vi "Target Sender.vi"() -> ()   [LabVIEW 2013]
doc: "This example demonstrates how to handle communications with multiple servers at once. Each server will ping the host over UDP in order to establish a TCP connection. Once a TCP connection is established, the server and client work in a typical command based fashion. Instead of a single server to communicate with though, the client must handle multiple connections."
uses:
  vi.lib/NI/STM/TCP/TCP Connection Info.ctl
  vi.lib/NI/STM/SubVIs/MetaDataElement.ctl
  Target SubVIs/ClientConnectionStates.ctl
  vi.lib/NI/STM/TCP/TCP Read Options.ctl
  vi.lib/NI/STM/UDP/Set Meta Data (UDP Ref).vi
  vi.lib/NI/STM/UDP/Get Connection Reference (UDP).vi
  vi.lib/NI/STM/TCP/Set Meta Data (TCP Ref).vi
  vi.lib/NI/STM/TCP/Get Connection Reference (TCP).vi
  vi.lib/NI/STM/TCP/Write Message (TCP).vi
  vi.lib/NI/STM/UDP/Write Message (UDP).vi
  vi.lib/NI/STM/TCP/Read Meta Data (TCP Clst).vi
  vi.lib/NI/STM/TCP/Read Message (TCP).vi
  vi.lib/NI/STM/NI STM.lvlib
panel:
  out "Connection Info":T1
  out "Connected":bool
  out "Host IP Address":string
  out "Waveform Graph":dbl[](graph)
  out "My IP Address":string
  out "error  out":errorcluster
  in  "stop":bool
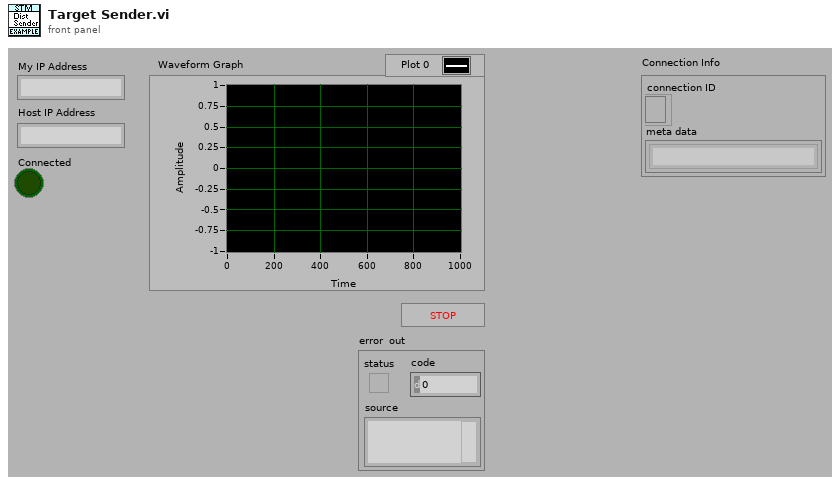
[diagram p1: front panel]
types:
  T1 = typedef "NI STM.lvlib/TCP Connection Info.ctl" = cluster{"connection ID":refnum<k5>, "meta data":T2[]}
  T2 = typedef "NI STM.lvlib/MetaDataElement.ctl" = string
  T3 = typedef "ClientConnectionStates.ctl" = enum16{"Init", "Ping Host", "Wait for Host Connection", "Read Meta Data", "Receive Commands", "Close Connection", "Shutdown"}
  T4 = typedef "NI STM.lvlib/TCP Read Options.ctl" = cluster{"ignore timeout error":bool, "timeout ms (1000)":i32}
  T5 = typedef "NI STM.lvlib/UDP Connection Info.ctl" = cluster{"connection ID":refnum<k16>, "meta data":T2[]}
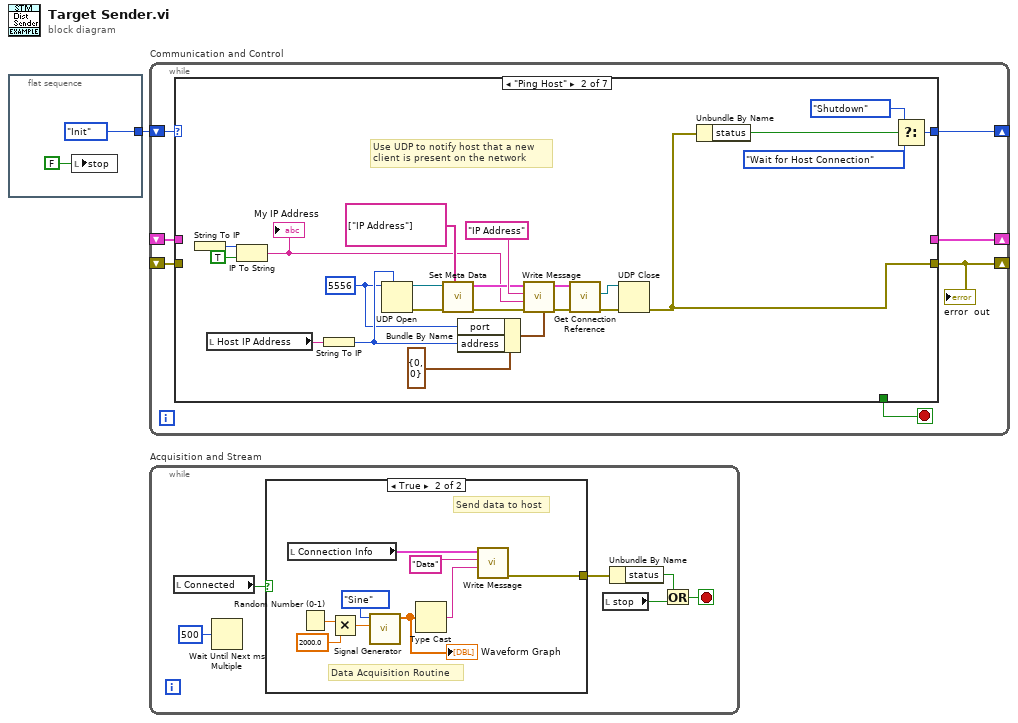
[diagram p0: block diagram]
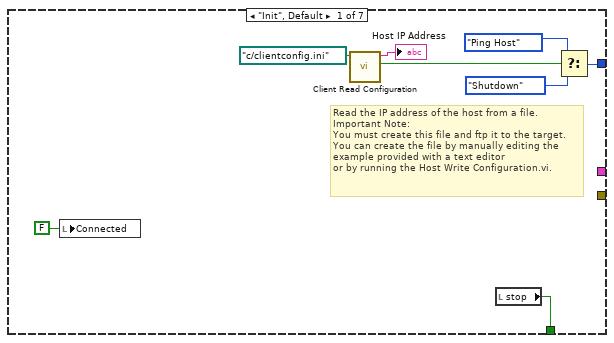
[diagram p2: hidden frame]
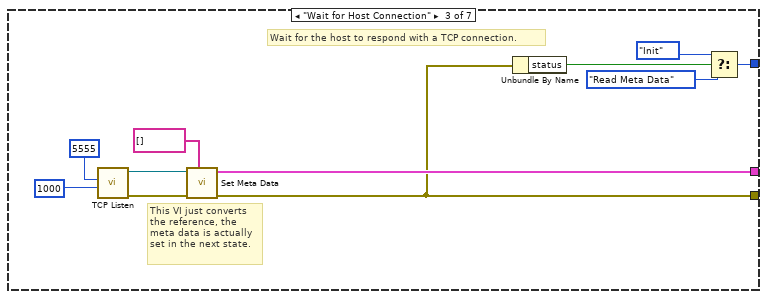
[diagram p3: hidden frame]
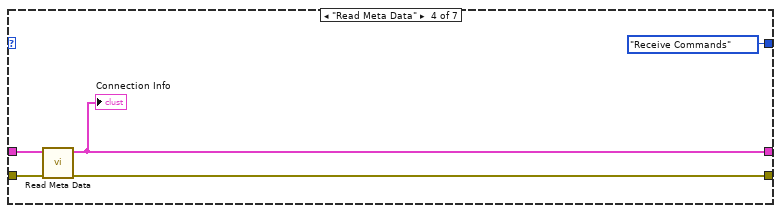
[diagram p4: hidden frame]
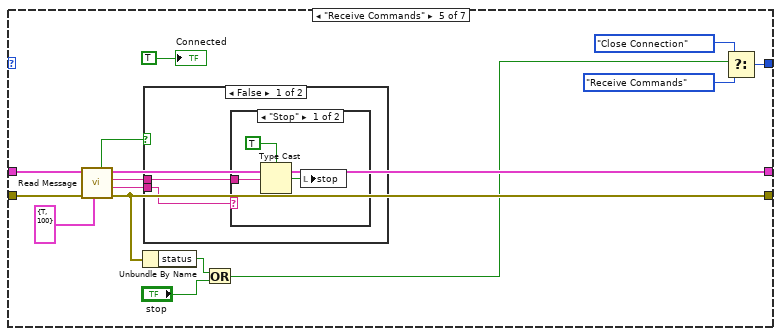
[diagram p5: hidden frame]
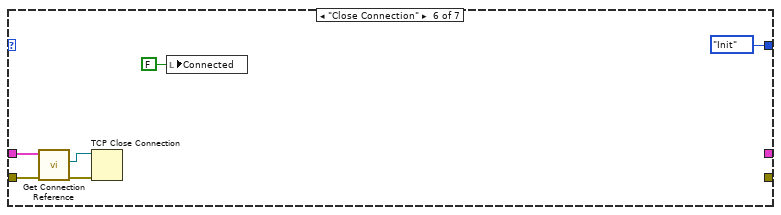
[diagram p8: hidden frame]
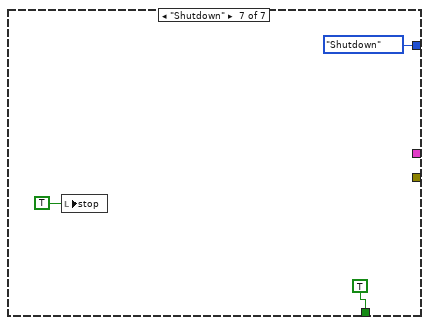
[diagram p9: hidden frame]
diagram:
  n1 = flat-sequence {
    tunnel: [ClientConnectionStates."Init" ("Connection States")] -> w1
    frame #0 {
      n2 = local write "stop"(FALSE ("stop")) -> ()
    }
  }
  n3 = while "Communication and Control" {
    shift-right: [w9] -> _
    shift-left: _ -> [w7]
    shift-right: [w8] -> _
    shift-left: w1 -> [w10]
    shift-right: [w5] -> _
    shift-left: _ -> [w6]
    stop <- w4 stop-if-true
    n4 = case shown="\"Ping Host\"" w10 {
      tunnel: [_ _ w44 w56 w70 _ _] -> w9
      tunnel: [w15 w37 w47 ClientConnectionStates."Receive Commands" ("Connection States") w60 ClientConnectionStates."Init" ("Connection States") ClientConnectionStates."Shutdown" ("Connection States")] -> w8
      tunnel: w7 -> [_ _ _ w57 w72 w79 _]
      tunnel: [_ w40 w43 w54 w69 _ _] -> w5
      tunnel: w6 -> [_ _ _ w55 w71 w81 _]
      tunnel: [w14 _ _ _ _ _ TRUE] -> w4
      frame "Init", Default {
        # "Read the IP address of the host from a file.\nImportant Note:\nYou must create this file and ftp it to the target.\nYou can create the file by manually editing the\nexample provided with a text editor\nor by running the Host Write Configuration.vi."
        n5 = local write "Connected"(FALSE ("Connected")) -> ()
        n6 = call "Client Read Configuration.vi"("configuration file path"=path "c:/clientconfig.ini") -> ("valid data"=w13:bool, "Host IP Address"=→"Host IP Address":string)  [unwired: 8 in, 1 out]
        n7 = local read "stop"() -> (w14:bool)
        n8 = Select(t=ClientConnectionStates."Ping Host" ("Connection States"), s=w13, f=ClientConnectionStates."Shutdown" ("Connection States")) -> (s? t:f=w15:T3)
      }
      frame "Ping Host" {
        w29 = u16 5556 ("port")
        # "Use UDP to notify host that a new client is present on the network"
        n9 = String To IP() -> (0:w20:u32)  [unwired: 1 out]
        n10 = local read "Host IP Address"() -> (w41:string)
        n11 = IP To String(1:TRUE ("dot notation? (F)"), 2:w20) -> (0:w19:string)
        "My IP Address" <- w19
        n12 = String To IP(1:w41) -> (0:w30:u32)
        n13 = UDP Open(7:w30, 11:w29) -> (port=w32:refnum<k16>, 0:w34:errorcluster)  [unwired: 3 in, 1 out]
        n14 = call-poly "Set Meta Data.vi"("meta data"=T2[] ["IP Address"] ("Meta data"), "error in"=w34, "connection ID"=w32) -> ("error out"=w33:errorcluster, "connection info out"=w31:T5)  [unwired: 7 in]
        n15 = Bundle By Name(cluster=cluster{"address":u32, "port":u16} {"address"=0, "port"=0} ("Address"), "port"=w29, "address"=w30) -> (w27:cluster{"address":u32, "port":u16})
        n16 = call-poly "Write Message.vi"("address"=w27, "error in"=w33, "data"=w19, "name"="IP Address" ("Name"), "connection info in"=w31) -> ("error out"=w26:errorcluster, "connection info out"=w24:T5)  [unwired: 5 in]
        n17 = call-poly "Get Connection Reference.vi"("error in"=w26, "connection info in"=w24) -> ("error out"=w25:errorcluster, "connection ID"=w23:refnum<k16>)  [unwired: 7 in, 1 out]
        n18 = UDP Close(connection ID=w23, 8:w25) -> (error out=w40:errorcluster)  [unwired: 1 out]
        n19 = Unbundle By Name(w40) -> ("status"=w38:bool)
        n20 = Select(t=ClientConnectionStates."Shutdown" ("Connection States"), s=w38, f=ClientConnectionStates."Wait for Host Connection" ("Connection States")) -> (s? t:f=w37:T3)
      }
      frame "Wait for Host Connection" {
        # "This VI just converts \nthe reference, the \nmeta data is actually \nset in the next state."
        # "Wait for the host to respond with a TCP connection."
        n21 = call <vilib>:"TCP Listen.vi"("timeout ms (wait forever: -1)"=1000, "port"=u16 5555) -> ("error out"=w45:errorcluster, "connection ID"=w46:refnum<k5>)  [unwired: 5 in, 3 out]
        n22 = call-poly "Set Meta Data.vi"("meta data"=T2[] [] ("Meta data"), "error in"=w45, "connection ID"=w46) -> ("error out"=w43:errorcluster, "connection info out"=w44:T1)  [unwired: 7 in]
        n23 = Unbundle By Name(w43) -> ("status"=w50:bool)
        n24 = Select(t=ClientConnectionStates."Init" ("Connection States"), s=w50, f=ClientConnectionStates."Read Meta Data" ("Connection States")) -> (s? t:f=w47:T3)
      }
      frame "Read Meta Data" {
        n25 = call-poly "Read Meta Data.vi"("error in"=w55, "connection info in"=w57) -> ("error out"=w54:errorcluster, "connection info out"=w56:T1)  [unwired: 7 in, 1 out]
        "Connection Info" <- w56
      }
      frame "Receive Commands" {
        n26 = call-poly "Read Message.vi"("options"=T4 {"ignore timeout error"=TRUE, "timeout ms (1000)"=100} ("Options"), "error in"=w71, "connection info in"=w72) -> ("error out"=w69:errorcluster, "name"=w66:T2, "data string"=w65:string, "connection info out"=w70:T1, "timed out?"=w64:bool)  [unwired: 3 in, 1 out]
        n27 = Unbundle By Name(w69) -> ("status"=w68:bool)
        n28 = case shown="False" w64 {
          tunnel: w66 -> [w73 _]
          tunnel: w65 -> [w74 _]
          frame False {
            n29 = case shown="\"Stop\"" w73 {
              tunnel: w74 -> [w77 _]
              frame "Stop" {
                n30 = Type Cast(type=TRUE, x=w77) -> (*(type *) &x=w76:bool)
                n31 = local write "stop"(w76) -> ()
              }
              frame Default {
              }
            }
          }
          frame True {
          }
        }
        n32 = Or(x=w68, y="stop") -> (x .or. y?=w63:bool)
        n33 = Select(t=ClientConnectionStates."Close Connection" ("Connection States"), s=w63, f=ClientConnectionStates."Receive Commands" ("Connection States")) -> (s? t:f=w60:T3)
        "Connected" <- TRUE
      }
      frame "Close Connection" {
        n34 = call-poly "Get Connection Reference.vi"("error in"=w81, "connection info in"=w79) -> ("error out"=w78:errorcluster, "connection ID out"=w80:refnum<k5>)  [unwired: 7 in, 1 out]
        n35 = TCP Close Connection(connection ID=w80, error in (no error)=w78) -> ()  [unwired: 1 in, 2 out]
        n36 = local write "Connected"(FALSE ("Connected")) -> ()
      }
      frame "Shutdown" {
        n37 = local write "stop"(TRUE ("stop")) -> ()
      }
    }
    "error  out" <- w5
  }
  n38 = while "Acquisition and Stream" {
    stop <- w92 stop-if-true
    n39 = local read "Connected"() -> (w87:bool)
    n40 = Wait Until Next ms Multiple(millisecond multiple=u32 500) -> ()  [unwired: 1 out]
    n41 = case shown="True" w87 {
      tunnel: [_ w100] -> w88
      frame False {
      }
      frame True {
        # "Send data to host"
        # "Data Acquisition Routine"
        n42 = local read "Connection Info"() -> (w93:T1)
        n43 = Random Number (0-1)() -> (number: 0 to 1=w97:dbl)
        n44 = Multiply(x=w97, y=2000.0) -> (x*y=w95:dbl)
        n45 = call "Signal Generator.vi"("frequency"=w95, "Signal Type"=enum16{"Sine", "Square", "Triangle", "Sawtooth"}."Sine") -> ("Data"=w94:dbl[])  [unwired: 8 in, 1 out]
        "Waveform Graph" <- w94
        n46 = Type Cast(x=w94) -> (*(type *) &x=w98:string)  [unwired: 1 in]
        n47 = call-poly "Write Message.vi"("data"=w98, "name"="Data" ("Name"), "connection info in"=w93) -> ("error out"=w100:errorcluster)  [unwired: 7 in, 1 out]
      }
    }
    n48 = local read "stop"() -> (w90:bool)
    n49 = Unbundle By Name(w88) -> ("status"=w91:bool)
    n50 = Or(x=w91, y=w90) -> (x .or. y?=w92:bool)
  }
